vi "Product.vi"(8 "error in (no error)":errorcluster, 9 "index":u16, 10 "Item Names":string[][](array[string]), 11 "Cafe in":refnum<class "Cafe.lvclass">) -> (0 "error out":errorcluster, 3 "Cafe out":refnum<class "Cafe.lvclass">)   [LabVIEW 2020, in "Cafe.lvlib" / "Cafe.lvclass"]
uses:
  Cafe.lvclass
  C:/Program Files (x86)/National Instruments/LabVIEW 2020/vi.lib/ActorFramework/Actor/Actor.lvclass
  <vilib>/ActorFramework/Actor/Actor.lvclass/Actor.ctl
  Cafe.lvclass/Cafe.ctl
  UI Actor Messages/Actualiza MSG Msg/Actualiza MSG Msg.lvclass/Actualiza MSG Msg.ctl
  <vilib>/ActorFramework/Message Enqueuer/Message Enqueuer.lvclass/Message Enqueuer.ctl
  <vilib>/ActorFramework/Message Enqueuer/Enqueue.vi
  UI Actor Messages/Actualiza MSG Msg/Actualiza MSG Msg.lvclass
  C:/Program Files (x86)/National Instruments/LabVIEW 2020/vi.lib/ActorFramework/Message/Message.lvclass
  <vilib>/ActorFramework/Message Priority Queue/Priority Enqueue.vi
  <vilib>/ActorFramework/Actor/Actor.lvclass
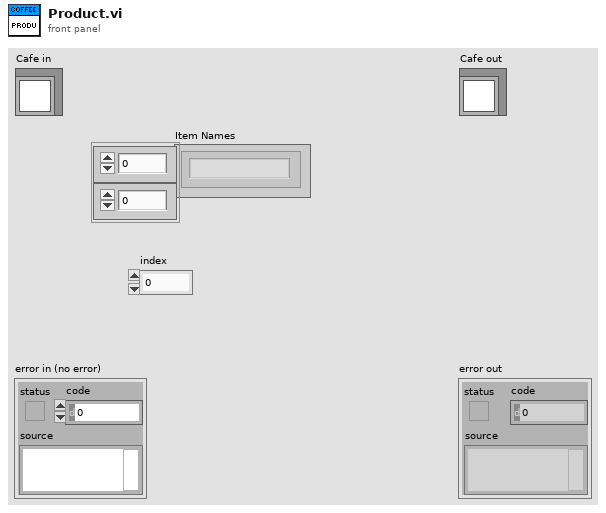
[diagram p1: front panel]
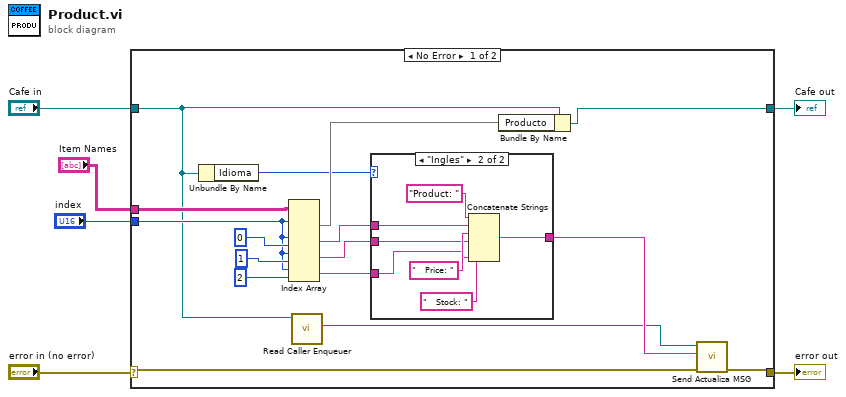
[diagram p0: block diagram]
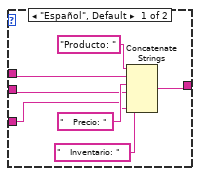
[diagram p2: hidden frame]
diagram:
  n1 = case shown="No Error" "error in (no error)" {
    selector: "error in (no error)" -> [w13 w38]
    tunnel: [w12 w38] -> w5
    tunnel: [w9 w37] -> w3
    tunnel: "Cafe in" -> [w8 w37]
    tunnel: "Item Names" -> [w11 _]
    tunnel: "index" -> [w10 _]
    frame No Error {
      n2 = Unbundle By Name(w8) -> ("Idioma"=w7:enum16{"Español", "Ingles"})
      n3 = Index Array(array=w11, index (row) #1=w10, index (row) #2=w10, index (col) #2=0 ("disabled index (col)"), index (row) #3=w10, index (col) #3=1 ("disabled index (col)"), index (row) #4=w10, index (col) #4=2 ("disabled index (col)")) -> (element #1=w15:string[], element #2=w16:string, element #3=w17:string, element #4=w18:string)  [unwired: 1 in]
      n4 = call <vilib>:"Read Caller Enqueuer.vi"("Actor"=w8) -> ("Caller Enqueuer"=w21:refnum<class "Message Enqueuer.lvclass">)  [unwired: 10 in]
      n5 = case shown="\"Ingles\"" w7 {
        tunnel: [w23 w33] -> w22
        tunnel: w18 -> [w24 w32]
        tunnel: w17 -> [w25 w31]
        tunnel: w16 -> [w26 w30]
        frame "Español", Default {
          n6 = Concatenate Strings("Producto: " ("string"), w26, "   Precio: " ("string"), w25, "   Inventario: " ("string"), w24) -> (w23:string)
        }
        frame "Ingles" {
          n7 = Concatenate Strings("Product: " ("string"), w30, "   Price: " ("string"), w31, "   Stock: " ("string"), w32) -> (w33:string)
        }
      }
      n8 = Bundle By Name(cluster=w8, "Producto"=w15) -> (w9:refnum<class "Cafe.lvclass">)
      n9 = call "Send Actualiza MSG.vi"("error in (no error)"=w13, "MSG"=w22, "Message Enqueuer"=w21) -> ("error out"=w12:errorcluster)  [unwired: 7 in, 1 out]
    }
    frame Error {
    }
  }
  "error out" <- w5
  "Cafe out" <- w3
